vi "Clonable Heartbeat.vi"(11 "Module ID":i32=-1) -> ()   [LabVIEW 2018]
uses:
  Libraries/Clonable Unit/Clonable Unit.lvlib
panel:
  out "ms":u32
  out "x >= y?":bool
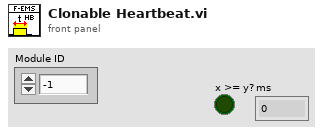
[diagram p1: front panel]
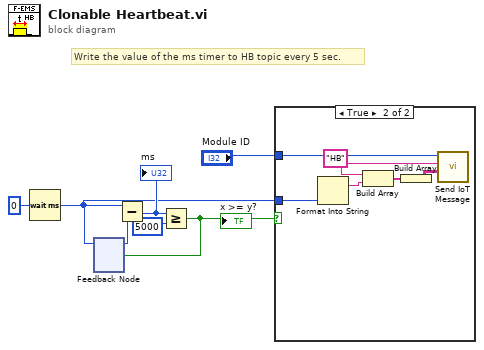
[diagram p0: block diagram]
diagram:
  # "Write the value of the ms timer to HB topic every 5 sec."
  n1 = Wait (ms)(milliseconds to wait=u32 0) -> (millisecond timer value=w2:u32)
  n2 = feedback #1() -> (w4:u32)  [unwired: 1 in]
  n3 = Subtract(x=w2, y=w4) -> (x-y=w7:u32)
  "ms" <- w7
  n4 = Greater Or Equal?(x=w7, y=u32 5000) -> (x >= y?=w5:bool)
  "x >= y?" <- w5
  n5 = feedback-in #1(w2, w5) -> ()
  n6 = case shown="True" w5 {
    tunnel: w2 -> [_ w13]
    tunnel: "Module ID" -> [_ w8]
    frame False {
    }
    frame True {
      w10 = "HB" ("Topic")
      n7 = Format Into String(w13) -> (resulting string=w12:string)  [unwired: 3 in, 1 out]
      n8 = Build Array(w10, w12) -> (w11:string[])
      n9 = Build Array(w11) -> (w9:string[][])
      n10 = call "Send IoT Message.vi"("Name Value Pairs"=w9, "Topic"=w10, "Module ID"=w8) -> ()  [unwired: 8 in, 1 out]
    }
  }
